vi "getTime.vi"(8 "error in (no error)":errorcluster, 11 "ScriptEvent.lvclass in":refnum<class "ScriptEvent.lvclass">) -> (0 "error out":errorcluster, 2 "time":dbl, 3 "ScriptEvent.lvclass out":refnum<class "ScriptEvent.lvclass">)   [LabVIEW 2011, in "Tools.lvlib" / "Scripting.lvlib" / "ScriptEvent.lvclass"]
uses:
  ScriptEvent.lvclass
  ScriptEvent.lvclass/ScriptEvent.ctl
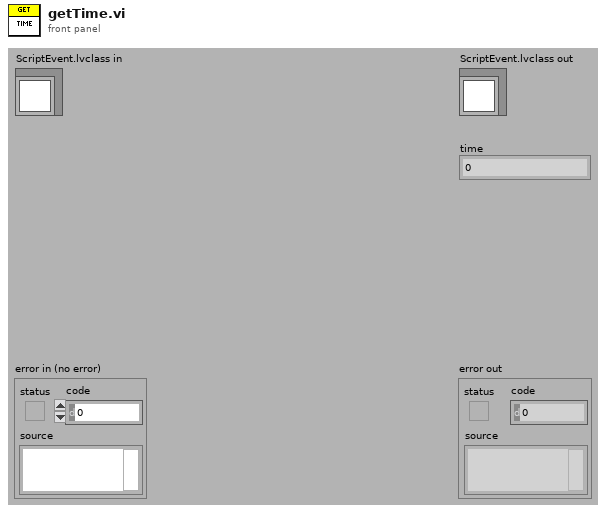
[diagram p1: front panel]
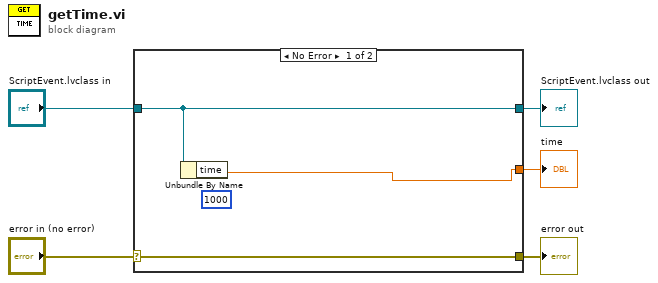
[diagram p0: block diagram]
diagram:
  n1 = case shown="No Error" "error in (no error)" {
    selector: "error in (no error)" -> [w8 w9]
    tunnel: [w8 w9] -> w4
    tunnel: [w7 w10] -> w2
    tunnel: "ScriptEvent.lvclass in" -> [w7 w10]
    tunnel: [w6 _] -> w1
    frame No Error {
      (unwired) 1000
      n2 = Unbundle By Name(w7) -> ("time"=w6:dbl)
    }
    frame Error {
    }
  }
  "error out" <- w4
  "ScriptEvent.lvclass out" <- w2
  "time" <- w1
